vi "Construct.vi"(1 "Acceleration":refnum<class "Vector2.lvclass">, 2 "Velocity":refnum<class "Vector2.lvclass">, 3 "Mass":sgl) -> (0 "PhysicsComponent out":refnum<class "PhysicsComponent.lvclass">)   [LabVIEW 2022 SP3, in "PhysicsComponent.lvclass"]
uses:
  PhysicsComponent.lvclass
  Math/Vector2/Vector2.lvclass
  PhysicsComponent.lvclass/PhysicsComponent.ctl
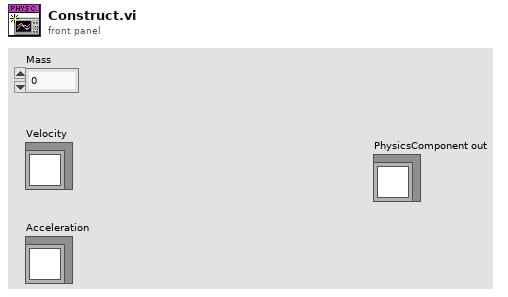
[diagram p1: front panel]
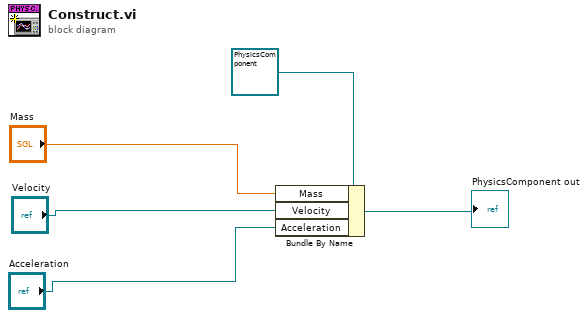
[diagram p0: block diagram]
diagram:
  n1 = Bundle By Name(cluster=refnum<class "PhysicsComponent.lvclass"> refnum ("PhysicsComponent.lvclass"), "Mass"="Mass", "Velocity"="Velocity", "Acceleration"="Acceleration") -> (→"PhysicsComponent out":refnum<class "PhysicsComponent.lvclass">)
